vi "anatomy.vi"() -> ()   [LabVIEW 8.6]
panel:
  out "error out":errorcluster
  out "function return 2":string
  # "anatomy.xlsx"
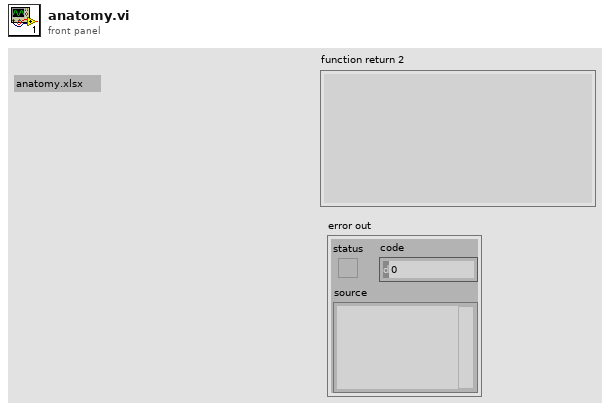
[diagram p1: front panel]
types:
  T1 = enum32{"invalid app kind", "Development System", "Run Time System", "Student Edition", "Embedded LabVIEW", "Evaluation", "Custom"}
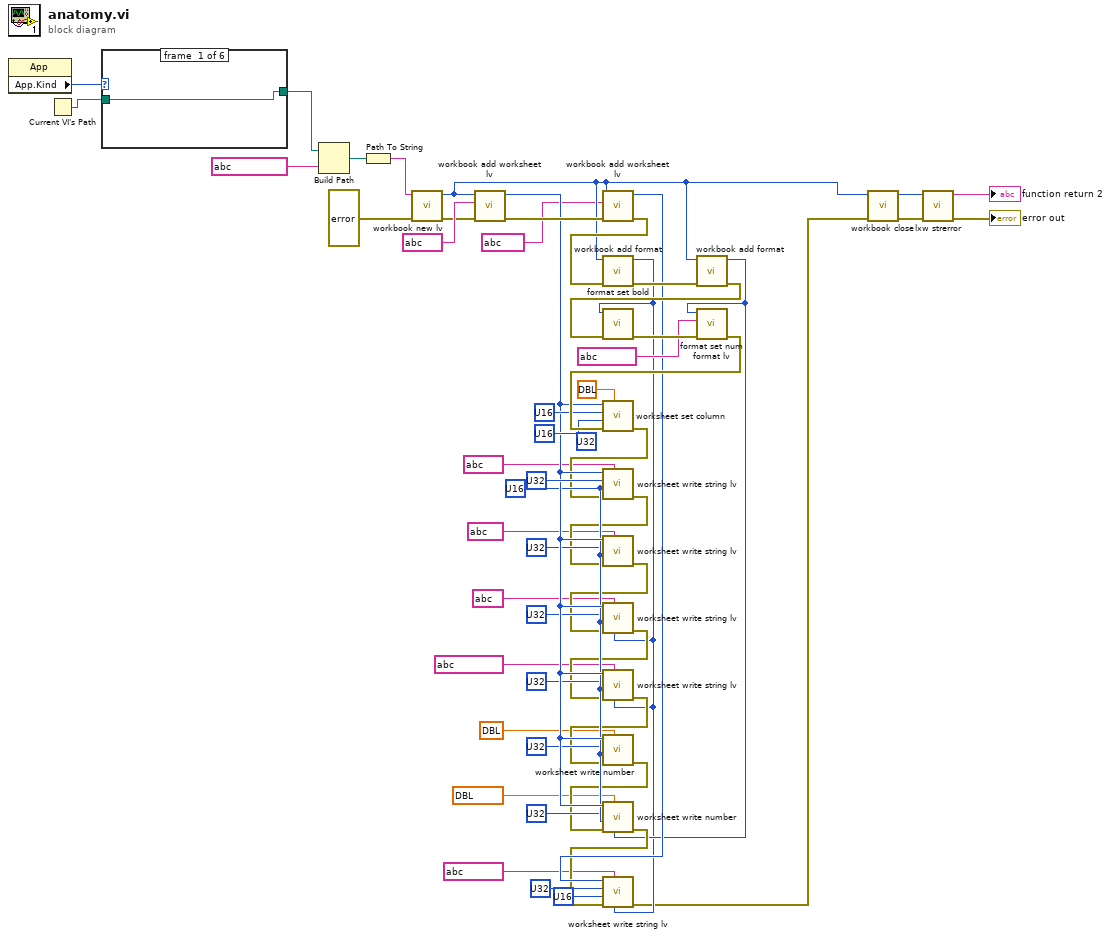
[diagram p0: block diagram]
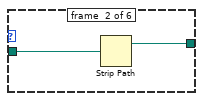
[diagram p2: hidden frame]
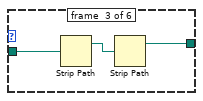
[diagram p3: hidden frame]
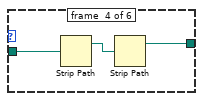
[diagram p4: hidden frame]
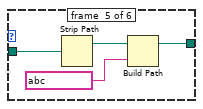
[diagram p5: hidden frame]
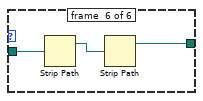
[diagram p6: hidden frame]
diagram:
  w28 = u16 ? ("col")
  (unwired) u32 ? ("format")
  n1 = property class="App"() -> ("App.Kind"=w53:T1)  [unwired: 2 in, 2 out]
  n2 = Current VI's Path() -> (path=w52:path)
  n3 = case shown="\"Evaluation\"" w53 {
    tunnel: w52 -> [w54 w56 w59 w62 w66 w69]
    tunnel: [w54 w55 w57 w60 w64 w67] -> w51
    frame #0 {
    }
    frame #1 {
      n4 = Strip Path(path=w56) -> (stripped path=w55:path)  [unwired: 1 out]
    }
    frame #2 {
      n5 = Strip Path(path=w59) -> (stripped path=w58:path)  [unwired: 1 out]
      n6 = Strip Path(path=w58) -> (stripped path=w57:path)  [unwired: 1 out]
    }
    frame #3 {
      n7 = Strip Path(path=w62) -> (stripped path=w61:path)  [unwired: 1 out]
      n8 = Strip Path(path=w61) -> (stripped path=w60:path)  [unwired: 1 out]
    }
    frame #4 {
      n9 = Strip Path(path=w66) -> (stripped path=w65:path)  [unwired: 1 out]
      n10 = Build Path(base path=w65, name or relative path=string ?) -> (appended path=w64:path)
    }
    frame #5 {
      n11 = Strip Path(path=w69) -> (stripped path=w68:path)  [unwired: 1 out]
      n12 = Strip Path(path=w68) -> (stripped path=w67:path)  [unwired: 1 out]
    }
  }
  n13 = Build Path(base path=w51, name or relative path=string ? ("filename")) -> (appended path=w42:path)
  n14 = Path To String(path=w42) -> (string=w41:string)
  n15 = call "workbook new lv.vi"("error in (no error)"=errorcluster ?, "filename"=w41) -> ("error out"=w48:errorcluster, "function return"=w2:u32)  [unwired: 8 in]
  n16 = call "workbook add worksheet lv.vi"("error in (no error)"=w48, "sheetname"=string ?, "workbook"=w2) -> ("error out"=w40:errorcluster, "function return"=w29:u32)  [unwired: 7 in]
  n17 = call "workbook add worksheet lv.vi"("error in (no error)"=w40, "sheetname"=string ?, "workbook"=w2) -> ("error out"=w39:errorcluster, "function return"=w21:u32)  [unwired: 7 in]
  n18 = call "workbook add format.vi"("error in (no error)"=w39, "workbook"=w2) -> ("error out"=w38:errorcluster, "function return"=w4:u32)  [unwired: 8 in]
  n19 = call "workbook add format.vi"("error in (no error)"=w38, "workbook"=w2) -> ("error out"=w37:errorcluster, "function return"=w5:u32)  [unwired: 8 in]
  n20 = call "format set bold.vi"("error in (no error)"=w37, "format"=w4) -> ("error out"=w36:errorcluster)  [unwired: 9 in]
  n21 = call "format set num format lv.vi"("error in (no error)"=w36, "num_format"=string ?, "format"=w5) -> ("error out"=w34:errorcluster)  [unwired: 8 in]
  n22 = call "worksheet set column.vi"("width"=dbl ?, "error in (no error)"=w34, "last_col"=u16 ?, "first_col"=u16 ?, "worksheet"=w29) -> ("error out"=w20:errorcluster)  [unwired: 5 in, 1 out]
  n23 = call "worksheet write string lv.vi"("string"=string ?, "error in (no error)"=w20, "col"=w28, "row"=u32 ?, "worksheet"=w29) -> ("error out"=w19:errorcluster)  [unwired: 5 in, 1 out]
  n24 = call "worksheet write string lv.vi"("string"=string ?, "error in (no error)"=w19, "col"=w28, "row"=u32 ?, "worksheet"=w29) -> ("error out"=w18:errorcluster)  [unwired: 5 in, 1 out]
  n25 = call "worksheet write string lv.vi"("format"=w4, "string"=string ?, "error in (no error)"=w18, "col"=w28, "row"=u32 ?, "worksheet"=w29) -> ("error out"=w17:errorcluster)  [unwired: 4 in, 1 out]
  n26 = call "worksheet write string lv.vi"("format"=w4, "string"=string ?, "error in (no error)"=w17, "col"=w28, "row"=u32 ?, "worksheet"=w29) -> ("error out"=w16:errorcluster)  [unwired: 4 in, 1 out]
  n27 = call "worksheet write number.vi"("number"=dbl ?, "error in (no error)"=w16, "col"=w28, "row"=u32 ?, "worksheet"=w29) -> ("error out"=w15:errorcluster)  [unwired: 5 in, 1 out]
  n28 = call "worksheet write number.vi"("format"=w5, "number"=dbl ?, "error in (no error)"=w15, "col"=w28, "row"=u32 ?, "worksheet"=w29) -> ("error out"=w14:errorcluster)  [unwired: 4 in, 1 out]
  n29 = call "worksheet write string lv.vi"("format"=w4, "string"=string ?, "error in (no error)"=w14, "col"=u16 ?, "row"=u32 ?, "worksheet"=w21) -> ("error out"=w3:errorcluster)  [unwired: 4 in, 1 out]
  n30 = call "workbook close.vi"("error in (no error)"=w3, "workbook"=w2) -> ("error out"=w44:errorcluster, "function return"=w46:u32)  [unwired: 8 in]
  n31 = call "lxw strerror.vi"("error in (no error)"=w44, "error_num"=w46) -> ("error out"=→"error out":errorcluster, "function return"=→"function return 2":string)  [unwired: 8 in]
